vi "függvényelso.vi"() -> ()   [LabVIEW 2011]
uses:
  <vilib>/express/express arith-compare/Formula/XNode/ExpressFormulaBlockNode.xnode
panel:
  in  "Tab Control":enum32{"tg(3a+0.8pi)", "x^(-3.2)", "lg(a+35)"}(tab)
  out "XY Graph":cluster{"Y":dbl[], "Y":dbl[]}[](graph)
  out "XY Graph 2":cluster{"Y":dbl[], "Y":dbl[]}[](graph)
  out "XY Graph 3":cluster{"Y":dbl[], "Y":dbl[]}[](graph)
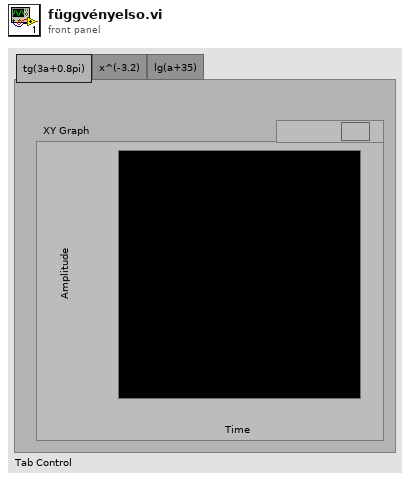
[diagram p1: front panel]
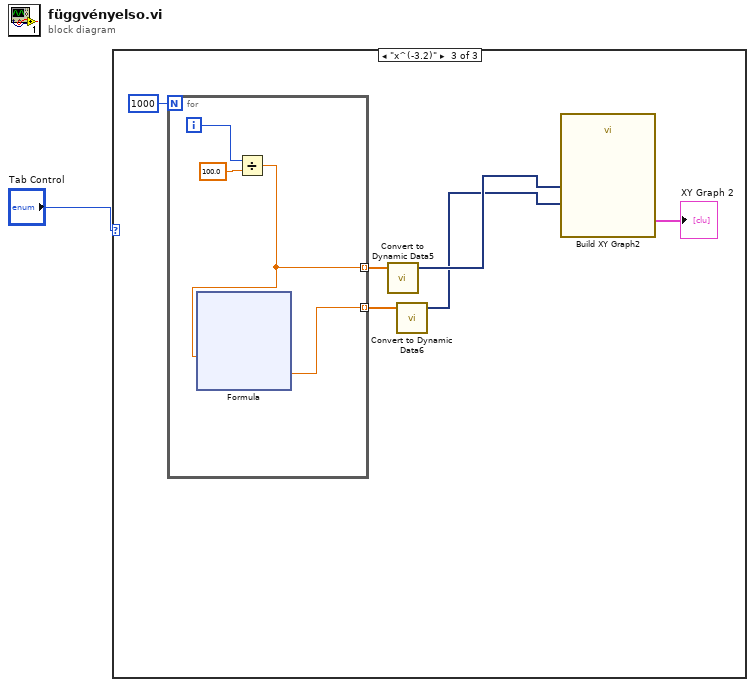
[diagram p0: block diagram]
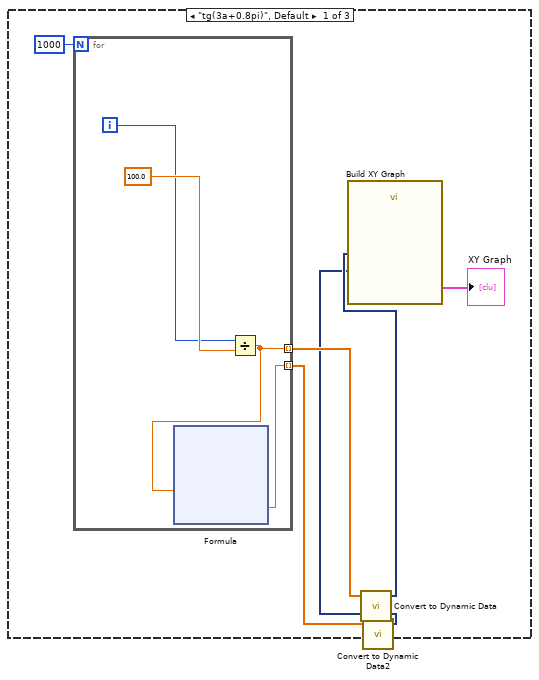
[diagram p2: hidden frame]
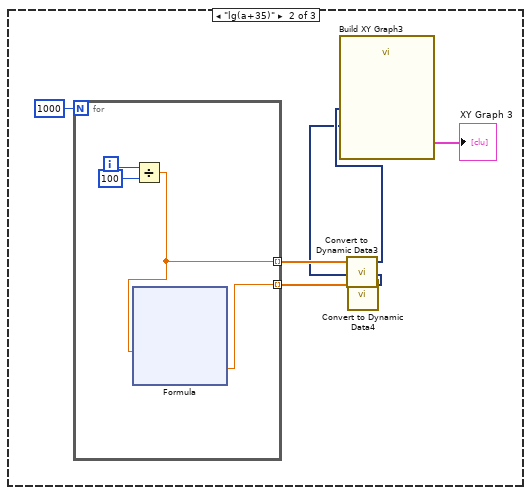
[diagram p3: hidden frame]
diagram:
  n1 = case shown="\"x^(-3.2)\"" "Tab Control" {
    frame "tg(3a+0.8pi)", Default {
      n2 = for {
        N: 1000 -> [_]
        tunnel: [w9] -> w6 mode=indexing
        tunnel: [w8] -> w5 mode=indexing
        i -> [w10]
        n3 = Divide(x=w10, y=100.0) -> (x/y=w9:dbl)
        n4 = xnode "Formula"("X1"=w9) -> ("Result"=w8:dbl)  [unwired: 1 in, 1 out]
      }
      n5 = call "Convert to Dynamic Data"("Array"=w6) -> ("Dynamic Data Type"=w3:dynamicdata)  [unwired: 3 in]
      n6 = call "Convert to Dynamic Data2"("Array"=w5) -> ("Dynamic Data Type"=w2:dynamicdata)  [unwired: 3 in]
      n7 = call "Build XY Graph"("Y Input"=w2, "X Input"=w3) -> ("XY Graph"=→"XY Graph":cluster{"Y":dbl[], "Y":dbl[]}[])  [unwired: 3 in, 6 out]
    }
    frame "lg(a+35)" {
      n8 = for {
        N: 1000 -> [_]
        tunnel: [w27] -> w24 mode=indexing
        tunnel: [w26] -> w23 mode=indexing
        i -> [w29]
        n9 = Divide(x=w29, y=100) -> (x/y=w27:dbl)
        n10 = xnode "Formula"("X1"=w27) -> ("Result"=w26:dbl)  [unwired: 1 in, 1 out]
      }
      n11 = call "Convert to Dynamic Data3"("Array"=w24) -> ("Dynamic Data Type"=w21:dynamicdata)  [unwired: 3 in]
      n12 = call "Convert to Dynamic Data4"("Array"=w23) -> ("Dynamic Data Type"=w20:dynamicdata)  [unwired: 3 in]
      n13 = call "Build XY Graph3"("Y Input"=w20, "X Input"=w21) -> ("XY Graph"=→"XY Graph 3":cluster{"Y":dbl[], "Y":dbl[]}[])  [unwired: 3 in, 6 out]
    }
    frame "x^(-3.2)" {
      n14 = for {
        N: 1000 -> [_]
        tunnel: [w45] -> w42 mode=indexing
        tunnel: [w44] -> w41 mode=indexing
        i -> [w46]
        n15 = Divide(x=w46, y=100.0) -> (x/y=w45:dbl)
        n16 = xnode "Formula"("X1"=w45) -> ("Result"=w44:dbl)  [unwired: 1 in, 1 out]
      }
      n17 = call "Convert to Dynamic Data5"("Array"=w42) -> ("Dynamic Data Type"=w39:dynamicdata)  [unwired: 3 in]
      n18 = call "Convert to Dynamic Data6"("Array"=w41) -> ("Dynamic Data Type"=w38:dynamicdata)  [unwired: 3 in]
      n19 = call "Build XY Graph2"("Y Input"=w38, "X Input"=w39) -> ("XY Graph"=→"XY Graph 2":cluster{"Y":dbl[], "Y":dbl[]}[])  [unwired: 3 in, 6 out]
    }
  }
